vi "Template Read Parameter File.vi"(6 "Import?":bool, 8 "error in (no error)":errorcluster, 10 "Alternate Path (\"\")":path, 11 "Template Record":T1) -> (0 "error out":errorcluster, 1 "Layout Files":string[](array[string]), 2 "Parameters":T2, 3 "updated Template Record":T1, 5 "estimate to complete (secs)":i32)   [LabVIEW 2011]
uses:
  Addons/internet/utils/keyedarr.llb/Keyed Array.ctl
  Template Record.ctl
  <vilib>/Utility/config.llb/Read Key (String).vi
  <vilib>/Utility/config.llb/NI_LVConfig.lvlib
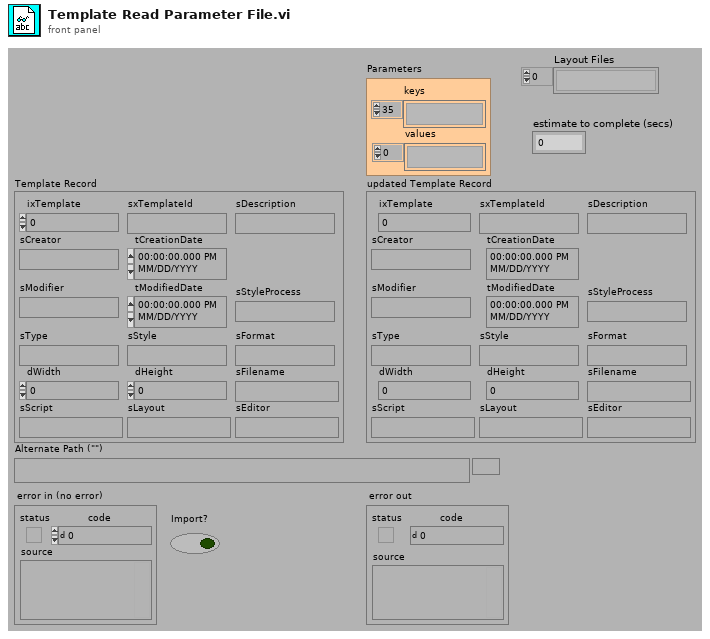
[diagram p1: front panel]
types:
  T1 = typedef "Template Record.ctl" = cluster{"ixTemplate":i32, "sxTemplateId":string, "sDescription":string, "sCreator":string, "tCreationDate":timestamp, "sModifier":string, "tModifiedDate":timestamp, "sType":string, "sStyle":string, "sFormat":string, "dWidth":dbl, "dHeight":dbl, "sFilename":string, "sScript":string, "sLayout":string, "sEditor":string, "sStyleProcess":string}
  T2 = typedef "Keyed Array.ctl" = cluster{"keys":string[], "values":string[]}
  T3 = typedef "NI_LVConfig.lvlib/Config Data RefNum.ctl" = refnum<k1>
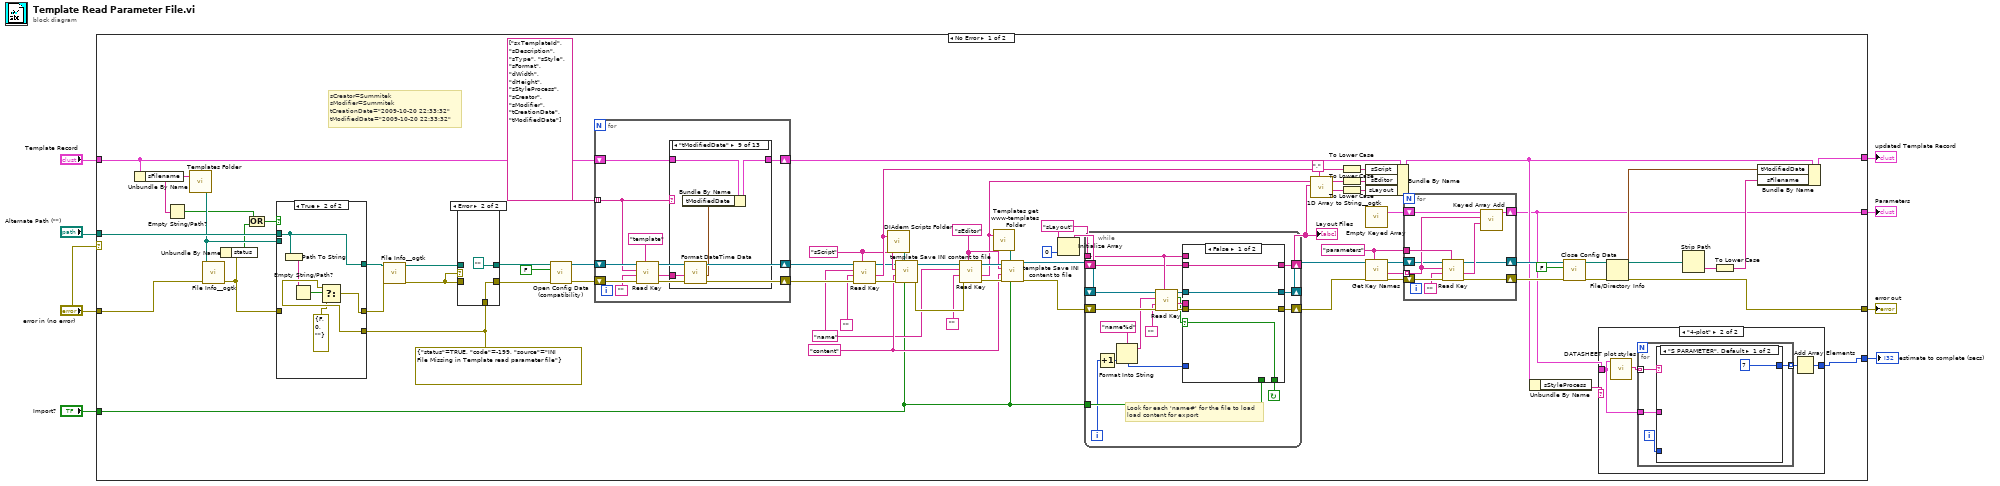
[diagram p0: block diagram]
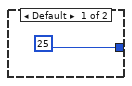
[diagram p2: hidden frame]
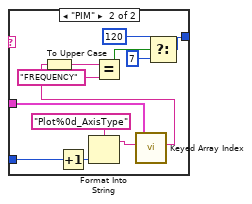
[diagram p3: hidden frame]
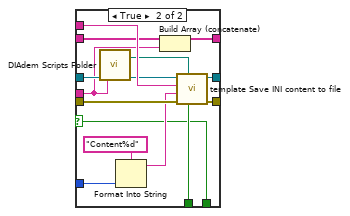
[diagram p5: hidden frame]
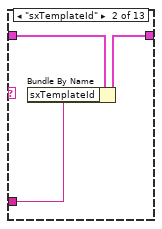
[diagram p8: hidden frame]
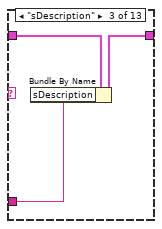
[diagram p9: hidden frame]
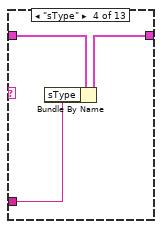
[diagram p10: hidden frame]
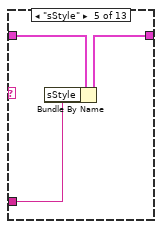
[diagram p11: hidden frame]
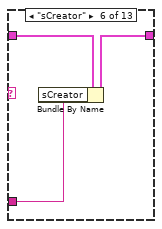
[diagram p12: hidden frame]
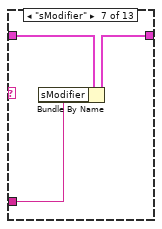
[diagram p13: hidden frame]
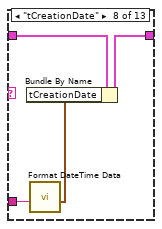
[diagram p14: hidden frame]
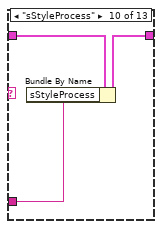
[diagram p15: hidden frame]
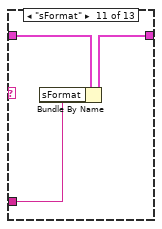
[diagram p16: hidden frame]
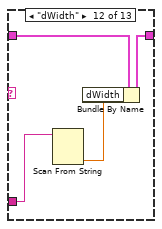
[diagram p17: hidden frame]
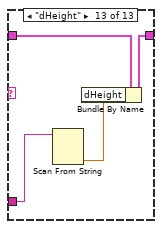
[diagram p18: hidden frame]
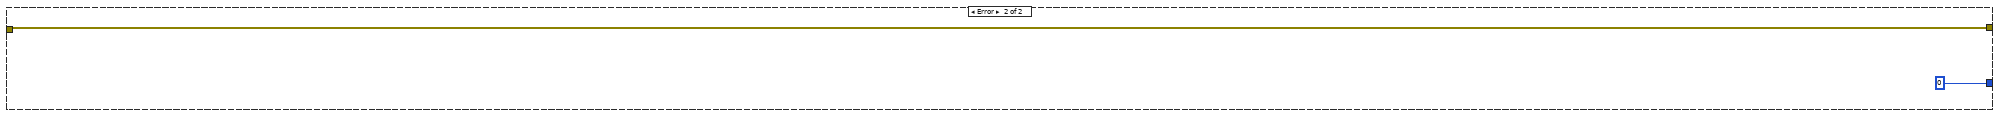
[diagram p19: hidden frame]
diagram:
  n1 = case shown="No Error" "error in (no error)" {
    tunnel: [w81 _] -> w8
    tunnel: [w14 _] -> w7
    tunnel: "Template Record" -> [w64 _]
    tunnel: "error in (no error)" -> [w53 w214]
    tunnel: "Alternate Path (\"\")" -> [w52 _]
    tunnel: "Import?" -> [w36 _]
    tunnel: [w35 w214] -> w3
    tunnel: [w13 0] -> w1
    frame No Error {
      w9 = errorcluster {"status"=TRUE, "code"=-199, "source"="INI File Missing in Template read parameter file"} ("error out")
      w31 = "sLayout" ("section")
      w48 = "sEditor" ("section")
      w40 = "content" ("section")
      w37 = "name" ("section")
      w57 = "sScript" ("section")
      w73 = "parameters" ("section")
      # "sCreator=Summitek\nsModifier=Summitek\ntCreationDate=\"2009-10-20 22:33:32\"\ntModifiedDate=\"2009-10-20 22:33:32\""
      n2 = Unbundle By Name(w64) -> ("sFilename"=w21:string)
      n3 = Empty String/Path?(string/path=w21) -> (empty?=w20:bool)
      n4 = call "Templates Folder.vi"("Relative Path (\"\")"=w21) -> ("Templates Folder"=w29:path)  [unwired: 2 out]
      n5 = call "File Info__ogtk.vi"("error in (no error)"=w53, "file"=w29) -> ("error out"=w19:errorcluster)  [unwired: 2 in, 4 out]
      n6 = Unbundle By Name(w19) -> ("status"=w18:bool)
      n7 = Or(x=w20, y=w18) -> (x .or. y?=w17:bool)
      n8 = case shown="True" w17 {
        tunnel: [w145 w149] -> w28
        tunnel: [w144 w151] -> w27
        tunnel: w52 -> [_ w151]
        tunnel: w29 -> [w144 _]
        tunnel: w19 -> [w145 _]
        tunnel: w9 -> [_ w148]
        frame False {
        }
        frame True {
          n9 = Path To String(path=w151) -> (string=w146:string)
          n10 = Empty String/Path?(string/path=w146) -> (empty?=w150:bool)
          n11 = Select(t=w148, s=w150, f=errorcluster {"status"=FALSE, "code"=0, "source"=""}) -> (s? t:f=w149:errorcluster)
        }
      }
      n12 = call "File Info__ogtk.vi"("error in (no error)"=w28, "file"=w27) -> ("error out"=w22:errorcluster, "file out"=w24:path)  [unwired: 2 in, 3 out]
      n13 = case shown="Error" w22 {
        tunnel: [w105 w106] -> w26
        tunnel: [w104 path ""] -> w25
        tunnel: w22 -> [w105 _]
        tunnel: w9 -> [_ w106]
        tunnel: w24 -> [w104 _]
        frame No Error {
        }
        frame Error {
        }
      }
      n14 = call <vilib>:"Open Config Data (compatibility).vi"("error in (no error)"=w26, "create file if necessary (T)"=FALSE, "configuration file path"=w25) -> ("error out"=w66:errorcluster, "refnum"=w65:T3)  [unwired: 6 in, 1 out]
      n15 = for {
        tunnel: string[] ["sxTemplateId", "sDescription", "sType", "sStyle", "sFormat", "dWidth", "dHeight", "sStyleProcess", "sCreator", "sModifier", "tCreationDate", "tModifiedDate"] -> [w154] mode=indexing
        shift-right: [w156] -> w41
        shift-left: w64 -> [w157]
        shift-right: [w159] -> w62
        shift-left: w66 -> [w161]
        shift-right: [w153] -> w63
        shift-left: w65 -> [w158]
        n16 = call-poly <vilib>:"Read Key.vi"("section"="template", "error in (no error)"=w161, "default value"="", "key"=w154, "refnum"=w158) -> ("error out"=w159:errorcluster, "value"=w152:string, "refnum out"=w153:T3)  [unwired: 1 in, 3 out]
        n17 = case shown="\"tModifiedDate\"" w154 {
          tunnel: w157 -> [w162 w165 w168 w171 w174 w177 w180 w184 w188 w191 w194 w198 w202]
          tunnel: [w162 w164 w167 w170 w173 w176 w179 w183 w187 w190 w193 w197 w201] -> w156
          tunnel: w152 -> [_ w163 w166 w169 w172 w175 w178 w182 w186 w189 w192 w196 w200]
          frame "unknown", Default {
          }
          frame "sxTemplateId" {
            n18 = Bundle By Name(cluster=w165, "sxTemplateId"=w163) -> (w164:T1)
          }
          frame "sDescription" {
            n19 = Bundle By Name(cluster=w168, "sDescription"=w166) -> (w167:T1)
          }
          frame "sType" {
            n20 = Bundle By Name(cluster=w171, "sType"=w169) -> (w170:T1)
          }
          frame "sStyle" {
            n21 = Bundle By Name(cluster=w174, "sStyle"=w172) -> (w173:T1)
          }
          frame "sCreator" {
            n22 = Bundle By Name(cluster=w177, "sCreator"=w175) -> (w176:T1)
          }
          frame "sModifier" {
            n23 = Bundle By Name(cluster=w180, "sModifier"=w178) -> (w179:T1)
          }
          frame "tCreationDate" {
            n24 = call "Format DateTime Data.vi"("DB String in"=w182) -> ("Timestamp out"=w181:timestamp)  [unwired: 10 out]
            n25 = Bundle By Name(cluster=w184, "tCreationDate"=w181) -> (w183:T1)
          }
          frame "tModifiedDate" {
            n26 = call "Format DateTime Data.vi"("DB String in"=w186) -> ("Timestamp out"=w185:timestamp)  [unwired: 10 out]
            n27 = Bundle By Name(cluster=w188, "tModifiedDate"=w185) -> (w187:T1)
          }
          frame "sStyleProcess" {
            n28 = Bundle By Name(cluster=w191, "sStyleProcess"=w189) -> (w190:T1)
          }
          frame "sFormat" {
            n29 = Bundle By Name(cluster=w194, "sFormat"=w192) -> (w193:T1)
          }
          frame "dWidth" {
            n30 = Scan From String(input string=w196) -> (output 1=w195:dbl)  [unwired: 3 in, 4 out]
            n31 = Bundle By Name(cluster=w198, "dWidth"=w195) -> (w197:T1)
          }
          frame "dHeight" {
            n32 = Scan From String(input string=w200) -> (output 1=w199:dbl)  [unwired: 3 in, 4 out]
            n33 = Bundle By Name(cluster=w202, "dHeight"=w199) -> (w201:T1)
          }
        }
      }
      n34 = call-poly <vilib>:"Read Key.vi"("section"=w57, "error in (no error)"=w62, "default value"="", "key"=w37, "refnum"=w63) -> ("error out"=w58:errorcluster, "value"=w60:string, "refnum out"=w56:T3)  [unwired: 1 in, 3 out]
      n35 = call "DIAdem Scripts Folder.vi"("Relative Path (\"\" - Folder)"=w60) -> ("Scripts Folder"=w59:path)  [unwired: 2 out]
      n36 = call "template Save INI content to file.vi"("Import?"=w36, "file"=w59, "error in"=w58, "key"=w40, "section"=w57, "refnum out"=w56) -> ("error out"=w49:errorcluster, "refnum out 2"=w46:T3)  [unwired: 4 out]
      n37 = call-poly <vilib>:"Read Key.vi"("section"=w48, "error in (no error)"=w49, "default value"="", "key"=w37, "refnum"=w46) -> ("error out"=w50:errorcluster, "value"=w42:string, "refnum out"=w51:T3)  [unwired: 1 in, 3 out]
      n38 = call "Templates get www-templates Folder.vi"("Relative Path (\"\")"=w42) -> ("WWW-templates Folder"=w47:path)  [unwired: 2 in]
      n39 = call "template Save INI content to file.vi"("Import?"=w36, "file"=w47, "error in"=w50, "key"=w40, "section"=w48, "refnum out"=w51) -> ("error out"=w34:errorcluster, "refnum out 2"=w33:T3)  [unwired: 4 out]
      n40 = Initialize Array(w31, 0 ("dimension size")) -> (w32:string[])
      n41 = while {
        tunnel: w31 -> [w124]
        shift-right: [w122] -> w38
        shift-left: w34 -> [w123]
        shift-right: [w121] -> w39
        shift-left: w33 -> [w125]
        tunnel: w36 -> [w120]
        shift-right: [w108] -> w12
        shift-left: w32 -> [w109]
        i -> [w113]
        stop <- w110 continue-if-true
        # "Look for each 'name#' for the file to load\nload content for export"
        n42 = Increment(x=w113) -> (x+1=w112:i32)
        n43 = Format Into String(format string="name%d" ("section"), w112) -> (resulting string=w114:string)  [unwired: 2 in, 1 out]
        n44 = call-poly <vilib>:"Read Key.vi"("section"=w124, "error in (no error)"=w123, "default value"="", "key"=w114, "refnum"=w125) -> ("error out"=w117:errorcluster, "value"=w118:string, "found?"=w111:bool, "refnum out"=w116:T3)  [unwired: 1 in, 2 out]
        n45 = case shown="False" w111 {
          selector: w111 -> [w129 w133]
          tunnel: w124 -> [_ w143]
          tunnel: [w127 w142] -> w122
          tunnel: [w128 w141] -> w121
          tunnel: w120 -> [_ w140]
          tunnel: w118 -> [_ w130]
          tunnel: w117 -> [w127 w138]
          tunnel: w116 -> [w128 w137]
          tunnel: w112 -> [_ w135]
          tunnel: [w129 w133] -> w110
          tunnel: w109 -> [w126 w132]
          tunnel: [w126 w131] -> w108
          frame False {
          }
          frame True {
            n46 = call "DIAdem Scripts Folder.vi"("Relative Path (\"\" - Folder)"=w130) -> ("Scripts Folder"=w139:path)  [unwired: 2 out]
            n47 = Format Into String(format string="Content%d" ("section"), w135) -> (resulting string=w134:string)  [unwired: 2 in, 1 out]
            n48 = Build Array (concatenate)(w132, w130) -> (w131:string[])
            n49 = call "template Save INI content to file.vi"("Import?"=w140, "file"=w139, "error in"=w138, "key"=w134, "section"=w143, "refnum out"=w137) -> ("error out"=w142:errorcluster, "refnum out 2"=w141:T3)  [unwired: 4 out]
          }
        }
      }
      "Layout Files" <- w12
      n50 = call "1D Array to String__ogtk.vi"("delimiter (Tab)"=",", "Array of Strings"=w12) -> ("delimited string"=w10:string)  [unwired: 9 in]
      n51 = To Lower Case(string=w60) -> (all lower case string=w61:string)
      n52 = To Lower Case(string=w42) -> (all lower case string=w43:string)
      n53 = To Lower Case(string=w10) -> (all lower case string=w23:string)
      n54 = Bundle By Name(cluster=w41, "sScript"=w61, "sEditor"=w43, "sLayout"=w23) -> (w16:T1)
      n55 = call "Empty Keyed Array.vi"() -> ("empty keyed array"=w71:T2)  [unwired: 3 out]
      n56 = call <vilib>:"Get Key Names.vi"("section"=w73, "error in (no error)"=w38, "refnum"=w39) -> ("error out"=w72:errorcluster, "key names"=w70:string[], "refnum out"=w68:T3)  [unwired: 6 out]
      n57 = for {
        tunnel: w73 -> [w212]
        shift-right: [w205] -> w14
        shift-left: w71 -> [w210]
        tunnel: w70 -> [w208] mode=indexing
        shift-right: [w203] -> w67
        shift-left: w68 -> [w204]
        shift-right: [w206] -> w69
        shift-left: w72 -> [w211]
        n58 = call-poly <vilib>:"Read Key.vi"("section"=w212, "error in (no error)"=w211, "default value"="", "key"=w208, "refnum"=w204) -> ("error out"=w206:errorcluster, "value"=w207:string, "refnum out"=w203:T3)  [unwired: 1 in, 3 out]
        n59 = call "Keyed Array Add.vi"("value"=w207, "key"=w208, "array in"=w210) -> ("array out"=w205:T2)  [unwired: 1 in, 3 out]
      }
      n60 = Unbundle By Name(w16) -> ("sStyleProcess"=w15:string)
      n61 = call <vilib>:"Close Config Data.vi"("error in (no error)"=w69, "write file if changed (T)"=FALSE, "refnum"=w67) -> ("error out"=w78:errorcluster, "file path"=w77:path)  [unwired: 7 out]
      n62 = case shown="\"4-plot\"" w15 {
        tunnel: [25 w84] -> w13
        tunnel: w14 -> [_ w83]
        frame Default {
        }
        frame "4-plot" {
          n63 = call "DATASHEET plot styles.vi"("parameters"=w83) -> ("styles"=w86:string[])  [unwired: 9 in, 1 out]
          n64 = for {
            tunnel: w86 -> [w90] mode=indexing
            tunnel: [w89] -> w85 mode=indexing
            tunnel: w83 -> [w87]
            i -> [w88]
            n65 = case shown="\"S PARAMETER\", Default" w90 {
              tunnel: [7 w96] -> w89
              tunnel: w88 -> [_ w101]
              tunnel: w87 -> [_ w99]
              frame "S PARAMETER", Default {
              }
              frame "PIM" {
                n66 = Increment(x=w101) -> (x+1=w103:i32)
                n67 = Format Into String(format string="Plot%0d_AxisType", w103) -> (resulting string=w100:string)  [unwired: 2 in, 1 out]
                n68 = call "Keyed Array Index.vi"("key"=w100, "array in"=w99) -> ("value"=w98:string)  [unwired: 2 in, 3 out]
                n69 = To Upper Case(1:w98) -> (0:w93:string)
                n70 = Equal?(x=w93, y="FREQUENCY" ("regular expression")) -> (x = y?=w92:bool)
                n71 = Select(t=120, s=w92, f=7) -> (s? t:f=w96:i32)
              }
            }
          }
          n72 = Add Array Elements(numeric array=w85) -> (sum=w84:i32)
        }
      }
      n73 = File/Directory Info(path=w77, error in=w78) -> (path out=w74:path, last mod=w54:timestamp, error out=w35:errorcluster)  [unwired: 4 out]
      n74 = Strip Path(path=w74) -> (name=w76:string)  [unwired: 1 out]
      n75 = To Lower Case(string=w76) -> (all lower case string=w75:string)
      n76 = Bundle By Name(cluster=w16, "tModifiedDate"=w54, "sFilename"=w75) -> (w81:T1)
    }
    frame Error {
    }
  }
  "error out" <- w3
  "Parameters" <- w7
  "updated Template Record" <- w8
  "estimate to complete (secs)" <- w1
